vi "Evaluate Function.vi"(1 "x":dbl, 3 "Function Reference":refnum<vi>) -> (0 "f(x)":dbl)   [LabVIEW 2020, in "Automatic Differentiation.lvlib"]
uses:
  Automatic Differentiation.lvlib
  classes/Dual/Dual.lvclass
  classes/Dual/Dual.lvclass/Dual.ctl
  9b1629ae-3de0-49eb-9b0a-cc9e581fb6c0.vi
  9b1629ae-3de0-49eb-9b0a-cc9e581fb6c0.vi/5957e011-cf56-4527-b6ed-13c3a4ca997b.vi
  classes/Dual/Write a.vi
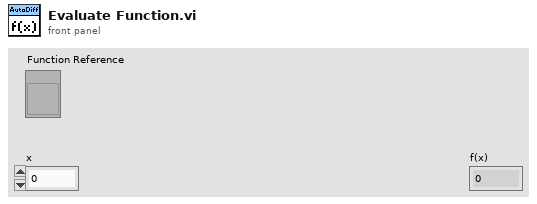
[diagram p1: front panel]
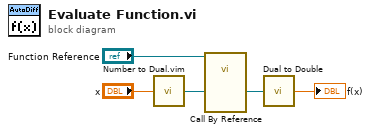
[diagram p0: block diagram]
diagram:
  n1 = call "Number to Dual.vim"("Number"="x") -> ("Dual"=w1:refnum<class "Dual.lvclass">)
  n2 = call-by-ref "?"(reference="Function Reference", "x"=w1) -> ("f(x)"=w4:refnum<class "Dual.lvclass">)  [unwired: 1 in, 2 out]
  n3 = call "Dual to Double.vi"("Dual"=w4) -> ("Double"=→"f(x)":dbl)
